vi "Sine_wave R3.vi"() -> ()   [LabVIEW 2018]
uses:
  <vilib>/measure/NI_MABase.lvlib
panel:
  in  "meas. time":dbl
  in  "dt FPGA":dbl
  out "Array":dbl[][](array[numeric])
  in  "Stop Button":bool
  in  "sampling info":cluster{"Fs":dbl, "#s":dbl}={"Fs"=1000.0, "#s"=1000.0} {"Fs" format="%.2p"}
  out "Waveform Graph":waveform(dbl)(graph)
  in  "amplitude\n[V]":dbl
  in  "Frequency \n[1/s]":dbl
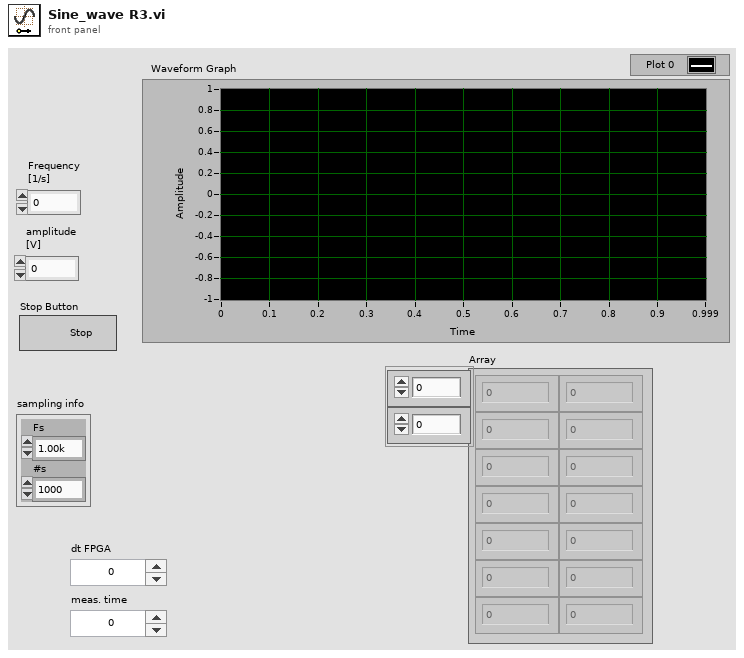
[diagram p1: front panel]
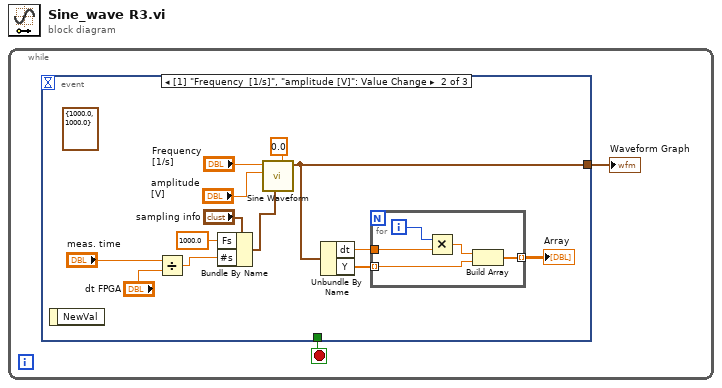
[diagram p0: block diagram]
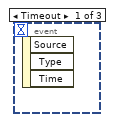
[diagram p2: hidden frame]
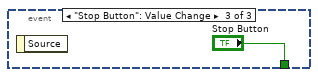
[diagram p3: hidden frame]
diagram:
  n1 = while {
    stop <- w2 stop-if-true
    n2 = event shown="[1] \"Frequency  [1/s]\", \"amplitude [V]\": Value Change" {
      selector: _ -> [_ _ _]
      dyn-events: _ -> [_ _ _]
      timeout: _ -> [_ _ _]
      tunnel: [_ w13 _] -> w1
      tunnel: [_ _ "Stop Button"] -> w2
      event Timeout {
        n3 = event-data() -> ()  [unwired: 1 in, 3 out]
      }
      event "Frequency \n[1/s]", "amplitude\n[V]": Value Change {
        (unwired) cluster{"Fs":dbl, "#s":dbl} {"Fs"=1000.0, "#s"=1000.0} ("sampling info")
        n4 = event-data() -> ()  [unwired: 1 in, 1 out]
        n5 = Divide(x="meas. time", y="dt FPGA") -> (x/y=w5:dbl)
        n6 = Bundle By Name(cluster="sampling info", "Fs"=1000.0, "#s"=w5) -> (w3:cluster{"Fs":dbl, "#s":dbl})
        n7 = call <vilib>:"Sine Waveform.vi"("offset"=0.0, "sampling info"=w3, "amplitude"="amplitude\n[V]", "frequency"="Frequency \n[1/s]") -> ("signal out"=w13:waveform(dbl))  [unwired: 6 in, 1 out]
        n8 = Unbundle By Name(w13) -> ("dt"=w10:dbl, "Y"=w11:dbl[])
        n9 = for {
          tunnel: w11 -> [w20] mode=indexing
          tunnel: w10 -> [w18]
          tunnel: [w16] -> w9 mode=indexing
          i -> [w19]
          n10 = Multiply(x=w19, y=w18) -> (x*y=w17:dbl)
          n11 = Build Array(w17, w20) -> (w16:dbl[])
        }
        "Array" <- w9
      }
      event "Stop Button": Value Change {
        n12 = event-data() -> ()  [unwired: 1 in, 1 out]
      }
    }
    "Waveform Graph" <- w1
  }
